vi "IMAQdx_setAttribute_Str.vi"(4 "error in (no error)":errorcluster, 5 "Value (String)":string, 6 "Attribute Name":string, 7 "IMAQdx Session":T1) -> (0 "error out":errorcluster, 1 "In Range?":bool, 3 "dup IMAQdx Session":T1)   [LabVIEW 2014, in "HGF_VisionTools.lvlib"]
doc: "This VI sets IMAQdx attribute value of type string."
uses:
  HGF_VisionTools.lvlib
  <resource>/objmgr/imaqdx.rc
  HGF_LVC/HGF_Auxiliary/HGF_Auxiliary.lvlib
  HGF_LVC/HGF_Auxiliary/Severity.ctl
  HGF_LVC/HGF_Auxiliary/ErrorCode.ctl
  <vilib>/userdefined/High Color/IMAQdx.ctl
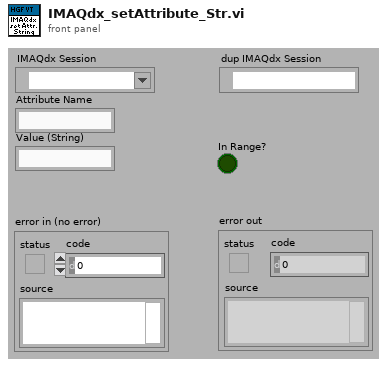
[diagram p1: front panel]
types:
  T1 = typedef "IMAQdx.ctl" = refnum<k21>
  T2 = typedef "HGF_Auxiliary.lvlib/ErrorCode.ctl" = enum32{"No error", "Function not supported.", "This VI is for friends only.", "Reference object aready exisits.", "Parameter out of range.", "Not a rendezvous.", "Invalid notifier reference.", "Invalid queue reference.", "Self-Test not supported.", "Reset not supported.", "IDN query not supported.", "Error query not supported.", "Incorrect addressee.", "Object already exists.", "No class name specified", "Driver not supported", "Attribute is not writable"}
  T3 = typedef "HGF_Auxiliary.lvlib/Severity.ctl" = enum16{"Info", "Warning", "Fault", "Error", "Fatal"}
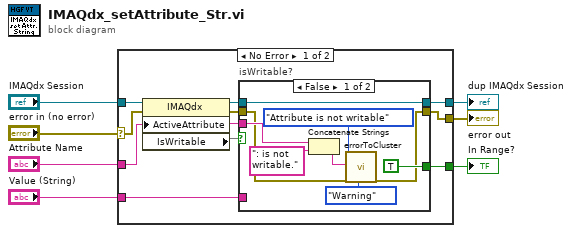
[diagram p0: block diagram]
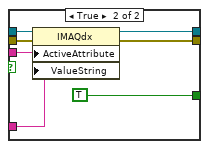
[diagram p2: hidden frame]
diagram:
  n1 = case shown="No Error" "error in (no error)" {
    selector: "error in (no error)" -> [w9 w34]
    tunnel: "IMAQdx Session" -> [w17 w35]
    tunnel: "Attribute Name" -> [w14 _]
    tunnel: "Value (String)" -> [w13 _]
    tunnel: [w12 w35] -> w4
    tunnel: [w11 w34] -> w3
    tunnel: [w10 _] -> w2
    frame No Error {
      n2 = property class="IMAQdx"(reference=w17, error in=w9, "ActiveAttribute"=w14) -> (reference out=w16:T1, error out=w15:errorcluster, "IsWritable"=w8)
      n3 = case "isWritable?" shown="False" w8 {
        tunnel: w16 -> [w26 w33]
        tunnel: w15 -> [w19 w32]
        tunnel: w14 -> [w20 w31]
        tunnel: w13 -> [_ w28]
        tunnel: [w26 w30] -> w12
        tunnel: [w18 w29] -> w11
        tunnel: [TRUE TRUE] -> w10
        frame False {
          n4 = Concatenate Strings(w20, ": is not writable." ("string")) -> (w21:string)
          n5 = call "errorToCluster.vi"("error code"=ErrorCode."Attribute is not writable", "error message (\"\")"=w21, "error in (no error)"=w19, "severity (Error)"=Severity."Warning") -> ("error out"=w18:errorcluster)  [unwired: 15 in]
        }
        frame True {
          n6 = property class="IMAQdx"(reference=w33, error in=w32, "ActiveAttribute"=w31, "ValueString"=w28) -> (reference out=w30:T1, error out=w29:errorcluster)
        }
      }
    }
    frame Error {
    }
  }
  "dup IMAQdx Session" <- w4
  "error out" <- w3
  "In Range?" <- w2
